vi "Test My JKI State Machine API.vi"() -> ()   [LabVIEW 2014, in "JKISM Example echo DQMH.lvlib"]
uses:
  JKISM Example echo DQMH.lvlib
  user.lib/_NEVSTOP/JKI State Machine ++/_Support/JKISMQ/_JKISMQFGV.vi
  user.lib/_NEVSTOP/JKI State Machine ++/JKI-State-Machine-Plus.lvlib
panel:
  out "Active Module":string[](array[string])
  in  "Select  Module":string(combo)
  out "Reply":string
  in  "X":dbl=1.0
  in  "wait for reply":bool=TRUE
  out "Reply Payload":dbl
  in  "Stop Module":bool
  in  "Start Module":bool
  in  "Test Do Something Else and Wait for Reply":bool
  in  "Hide Module Panel":bool
  in  "Show Module Panel":bool
  in  "Test Do Something Else":bool
  in  "Test Do Something":bool
  # "1. Support both Singleton and Cloneable , compare with DQMH Template\n2. Use the reply method -> as the replacement of status report in DQMH Template"
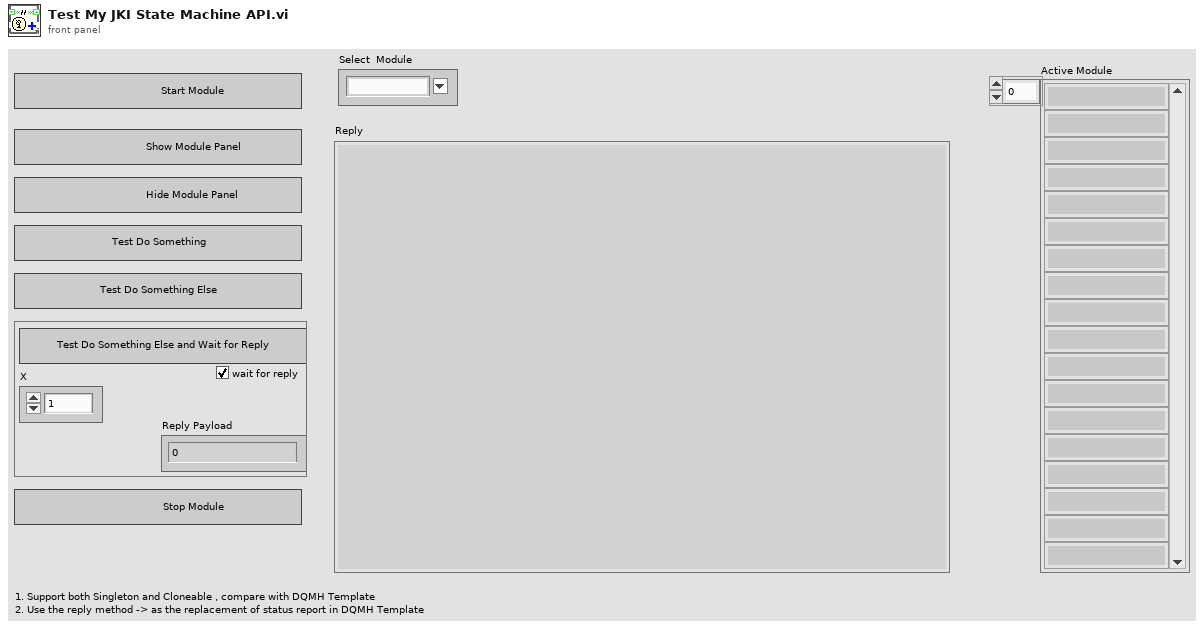
[diagram p1: front panel]
types:
  T1 = enum32{"Invalid", "Standard", "Closed", "Hidden", "Minimized", "Maximized"}
  T2 = enum32{"invalid app kind", "Development System", "Run Time System", "Student Edition", "Embedded LabVIEW", "Evaluation", "Custom"}
  T3 = cluster{"Core":cluster{"Current VI Reference":refnum<vi>, "Close Panel on Exit?":bool}, "Your Boolean data":bool, "Your string data":string, "Select  Module":refnum<vi>}
  T4 = cluster{"Current VI Reference":refnum<vi>, "Close Panel on Exit?":bool}
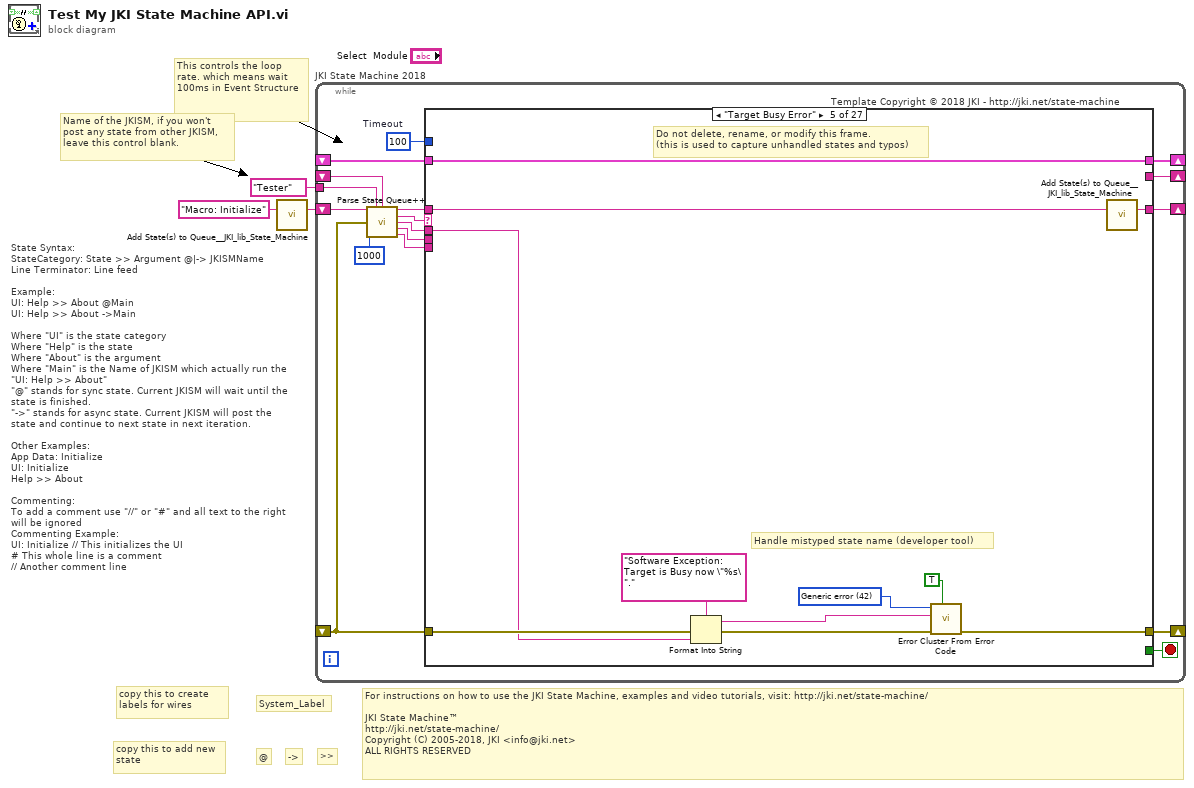
[diagram p0: block diagram]
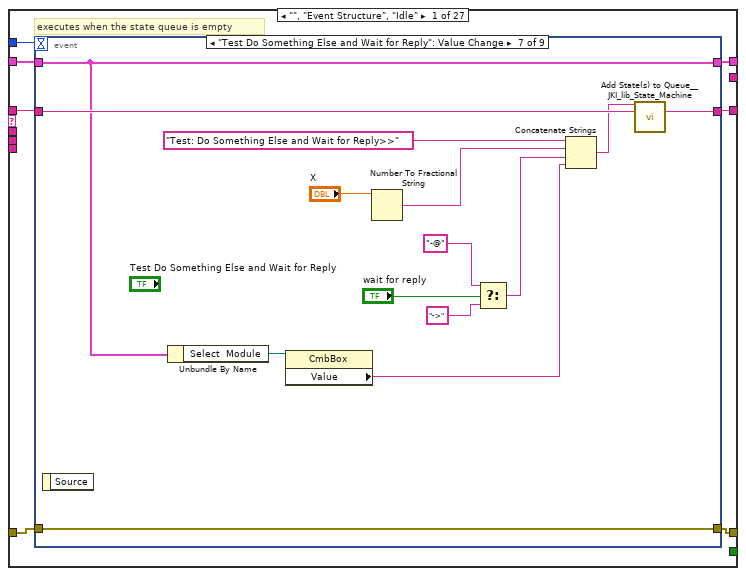
[diagram p2: hidden frame]
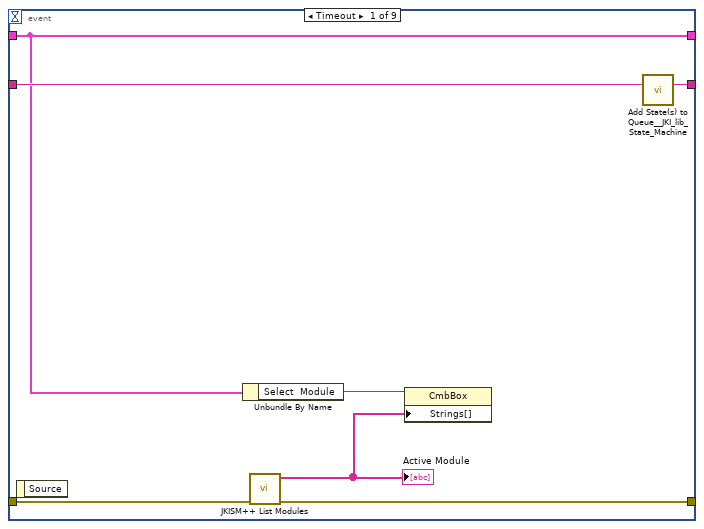
[diagram p3: hidden frame]
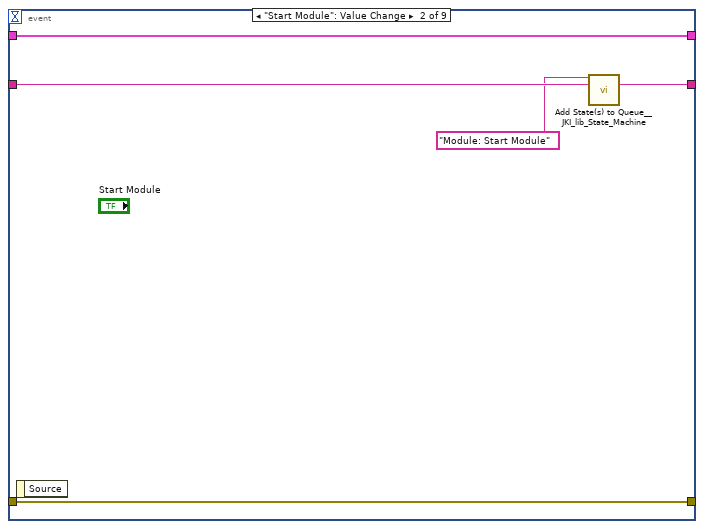
[diagram p4: hidden frame]
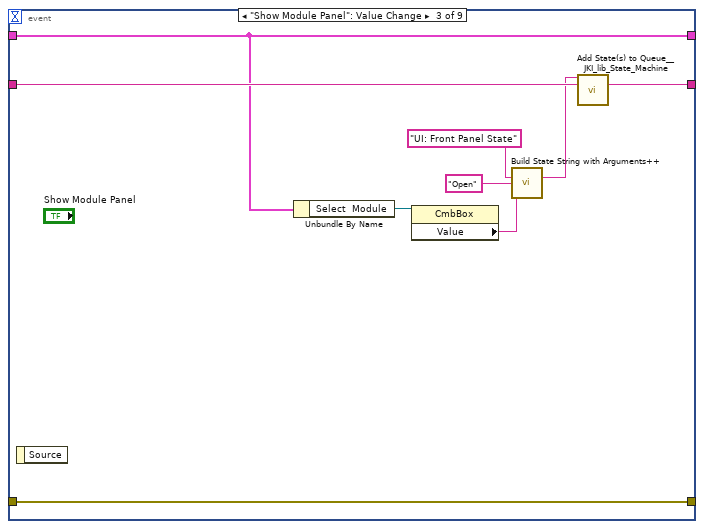
[diagram p5: hidden frame]
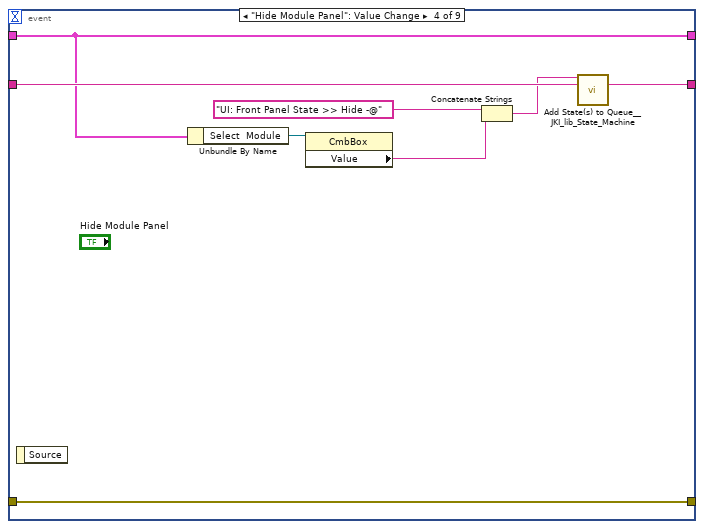
[diagram p6: hidden frame]
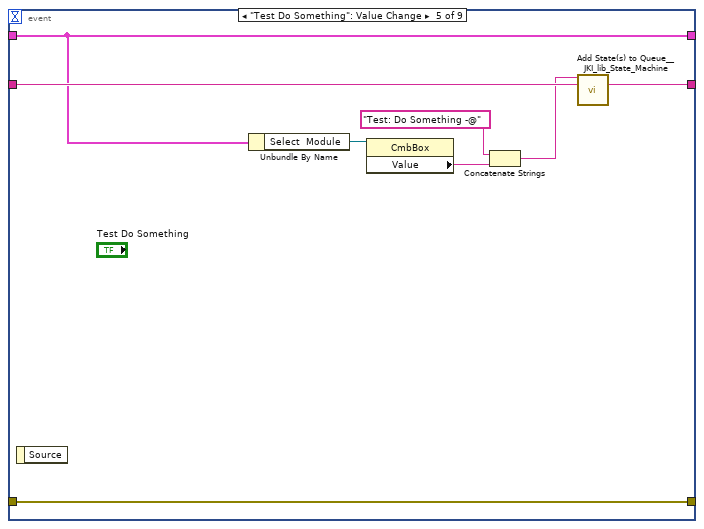
[diagram p7: hidden frame]
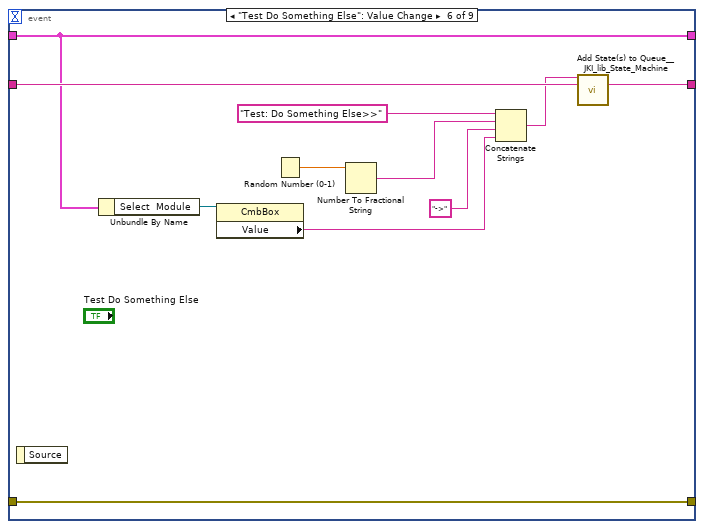
[diagram p8: hidden frame]
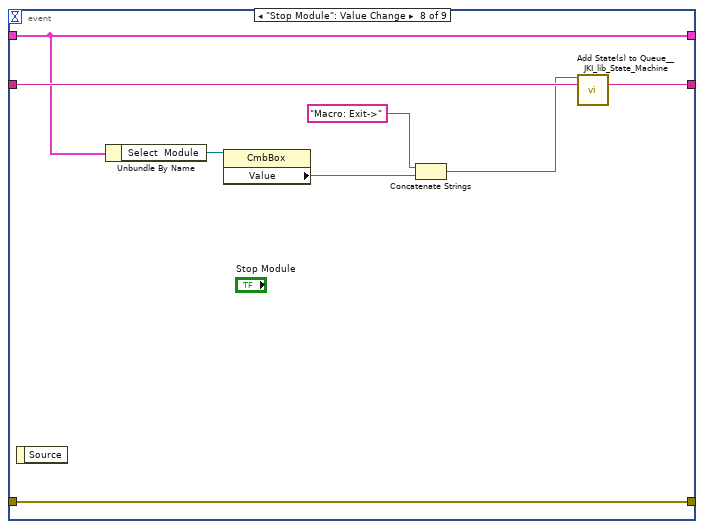
[diagram p9: hidden frame]
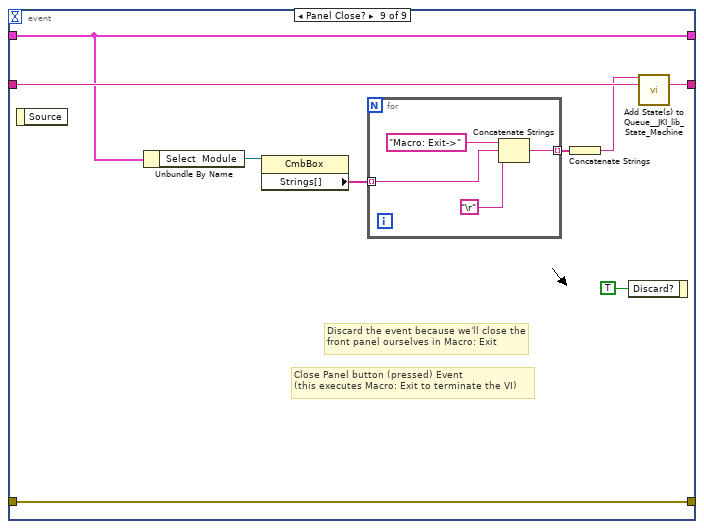
[diagram p10: hidden frame]
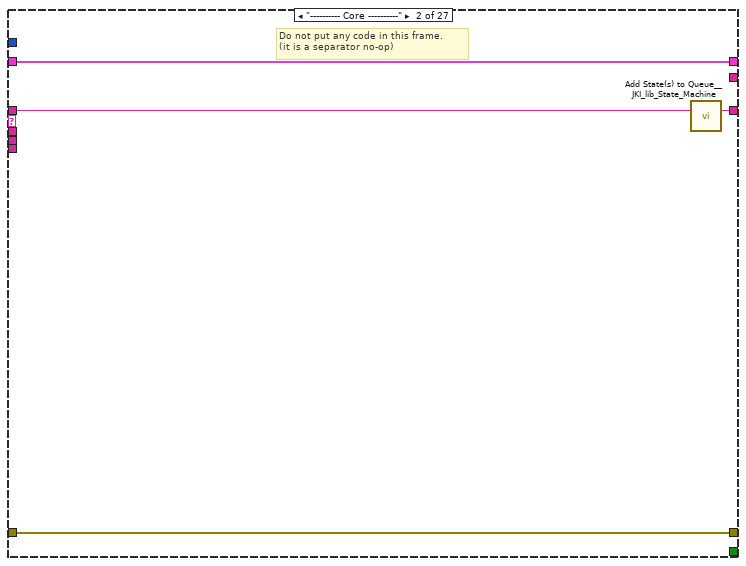
[diagram p11: hidden frame]
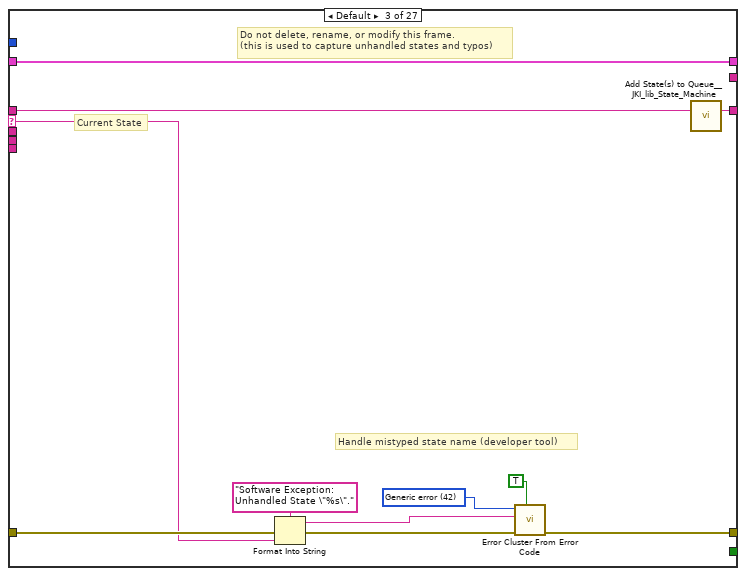
[diagram p12: hidden frame]
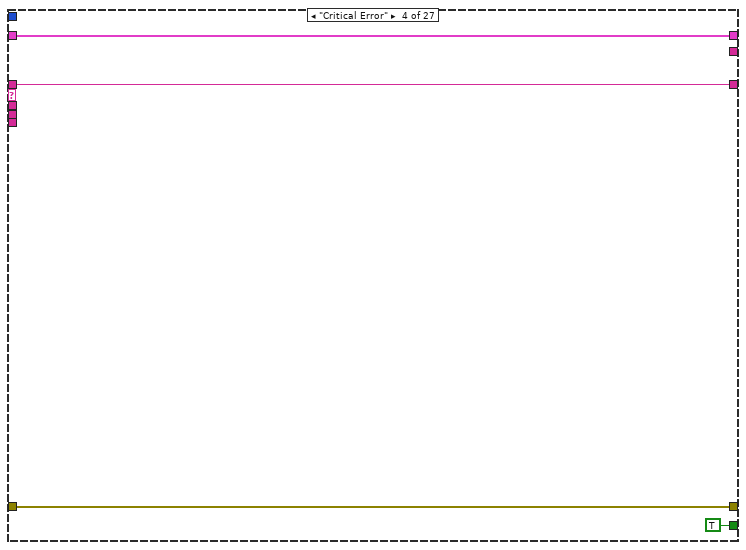
[diagram p13: hidden frame]
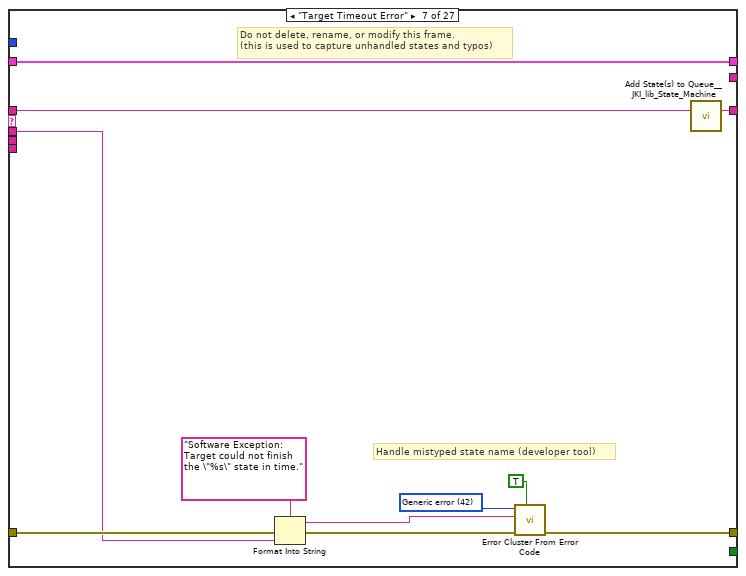
[diagram p15: hidden frame]
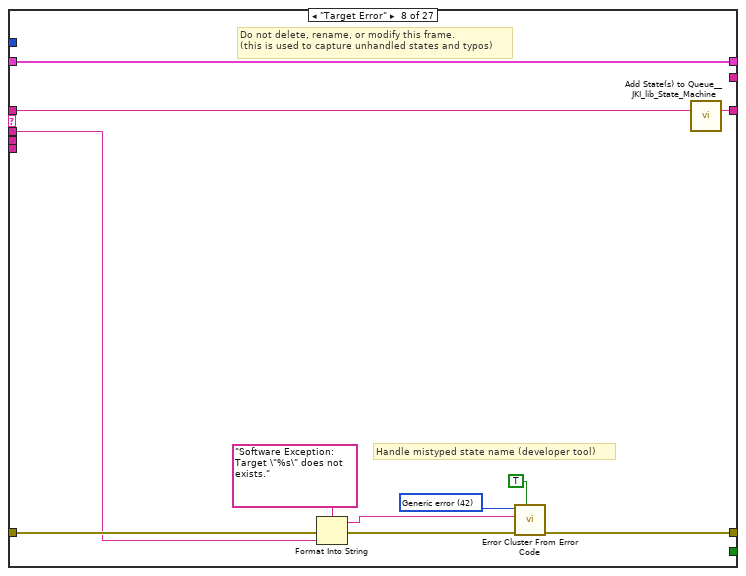
[diagram p16: hidden frame]
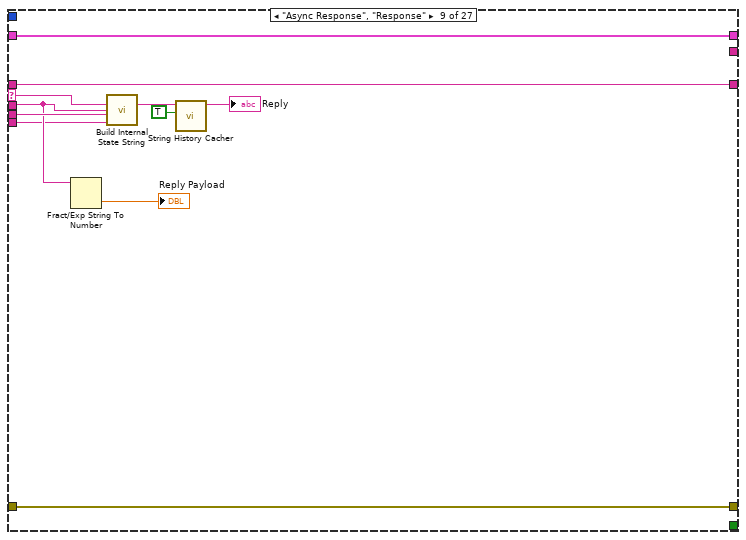
[diagram p17: hidden frame]
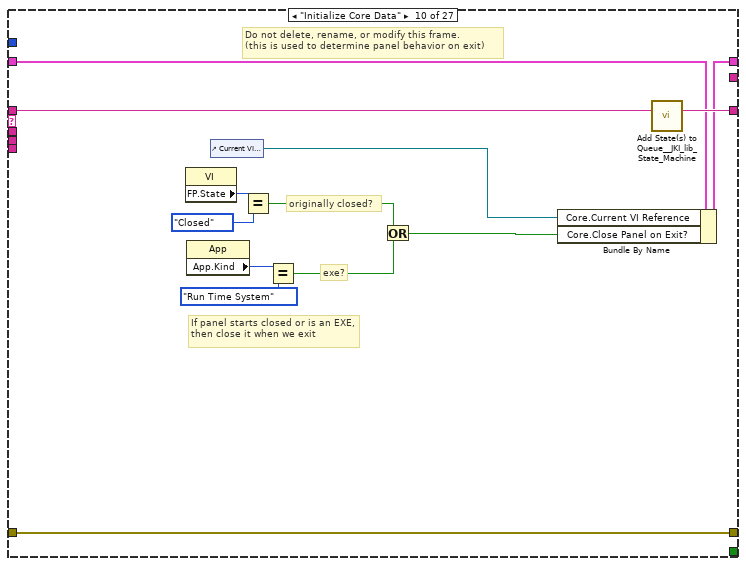
[diagram p18: hidden frame]
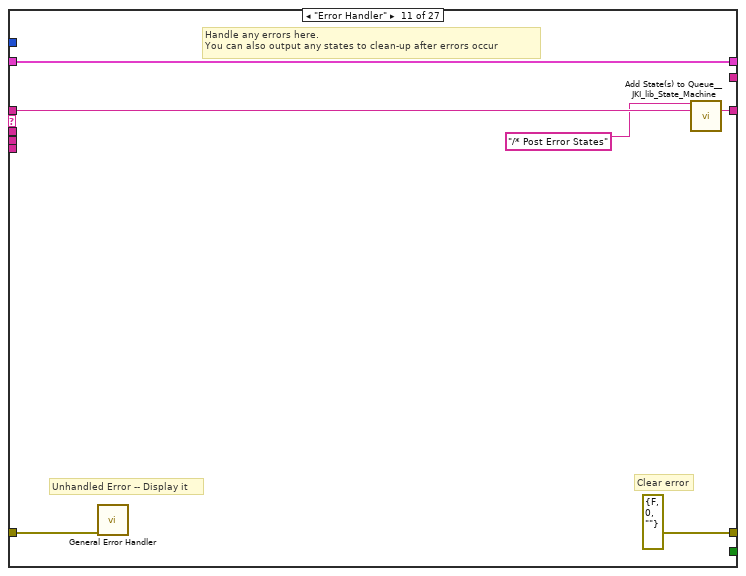
[diagram p19: hidden frame]
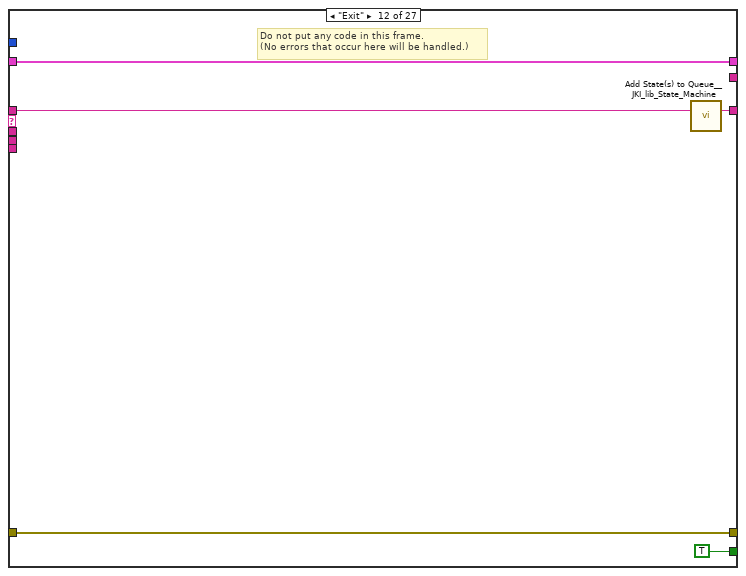
[diagram p20: hidden frame]
diagram:
  # "copy this to add new state"
  # ">>"
  # "->"
  # "@"
  # "Name of the JKISM, if you won't post any state from other JKISM,  leave this control blank."
  # "For instructions on how to use the JKI State Machine, examples and video tutorials, visit: http://jki.net/state-machine/\n\nJKI State Machine™\nhttp://jki.net/state-machine/\nCopyright (C) 2005-2018, JKI <info@jki.net>\nALL RIGHTS RESERVED"
  # "State Syntax:\nStateCategory: State >> Argument @|-> JKISMName\nLine Terminator: Line feed\n\nExample:\nUI: Help >> About @Main\nUI: Help >> About ->Main\n\nWhere \"UI\" is the state category\nWhere \"Help\" is the state\nWhere \"About\" is the argument\nWhere \"Main\" is the Name of JKISM which actually run the \"UI: Help >> About\"\n\"@\" stands for sync state. Current JKISM will wait until the state is finished.\n\"->\" stands for async state. Current JKISM will post the state and continue to next state in next iteration.\n\nOther Examples:\nApp Data: Initialize\nUI: Initialize\nHelp >> About\n\nCommenting:\nTo add a comment use \"//\" or \"#\" and all text to the right will be ignored\nCommenting Example:\nUI: Initialize // This initializes the UI\n# This whole line is a comment\n// Another comment line"
  # "copy this to create labels for wires"
  # "This controls the loop rate. which means wait 100ms in Event Structure"
  # "System_Label"
  n1 = call <vilib>:"Add State(s) to Queue__JKI_lib_State_Machine.vi"("State(s) in (\"\")"="Macro: Initialize") -> ("States Out"=w3:string)  [unwired: 14 in]
  n2 = while "JKI State Machine 2018" {
    shift-right: [w15] -> _
    shift-left: _ -> [w14]
    shift-right: [w18] -> _
    shift-left: _ -> [w12]
    shift-right: [w17] -> _
    shift-left: w3 -> [w19]
    tunnel: "Tester" ("Name(\"\" to use uuid)") -> [w8]
    shift-right: [w4] -> _
    shift-left: _ -> [w5]
    stop <- w16 stop-if-true
    w13 = 100  # Timeout
    # "Template Copyright © 2018 JKI - http://jki.net/state-machine"
    n3 = call "Parse State Queue++.vi"("State Queue"=w19, "Name(\"\" to use uuid)"=w8, "Response Arguments"=w5, "Error In (no error)"=w12, "Response Timeout(5000ms)"=1000 ("Response Timeout(1000ms)")) -> ("Remaining States"=w20:string, "Current State"=w11:string, "Arguments"=w10:string, "Argument - State"=w6:string, "From Who"=w9:string)  [unwired: 5 in, 1 out]
    n4 = case shown="\"Target Busy Error\"" w11 {
      selector: w11 -> [_ _ w115 _ _ _ _ _ w173 _ _ _ _ _ _ _ _ _ _ _ _ _ _ _ _ _ _]
      tunnel: w20 -> [w27 w114 w119 w128 w134 w142 w148 w159 w175 w189 w195 w200 w204 w212 w218 w222 w226 w232 w243 w312 w317 w327 w331 w335 w339 w341 w350]
      tunnel: w10 -> [_ _ _ _ w130 _ w144 w155 w169 _ _ _ _ _ _ _ _ w227 w237 _ _ _ _ _ _ _ _]
      tunnel: w14 -> [w25 w111 w117 w127 w132 w141 w146 w157 w174 w182 w192 w198 w201 _ w213 w219 w224 w230 w239 w309 w314 w324 w328 w332 w336 w340 w361]
      tunnel: [w24 w112 w121 w129 w136 w143 w150 w161 w176 w186 errorcluster {"status"=FALSE, "code"=0, "source"=""} ("error out") w197 w202 w209 w214 w220 w223 w228 w240 w310 w315 w325 w329 w333 w337 w342 w349] -> w18
      tunnel: w12 -> [w23 w112 w120 w129 w135 w143 w149 w160 w176 w186 w191 w197 w202 w209 w215 w220 w223 w229 w241 w310 w315 w325 w329 w333 w337 w342 w359]
      tunnel: [w26 w113 w118 w128 w133 w142 w147 w158 w175 w188 w194 w199 w203 w211 w217 w221 w225 w231 w242 w311 w316 w326 w330 w334 w338 w341 w350] -> w17
      tunnel: [_ _ _ TRUE _ _ _ _ _ _ _ TRUE _ _ _ _ _ _ _ _ _ _ _ _ _ _ _] -> w16
      tunnel: [w22 w111 w117 w127 w132 w141 w146 w157 w174 w187 w192 w198 w201 w210 w213 w219 w224 w230 w239 w309 w314 w324 w328 w332 w336 w340 w361] -> w15
      tunnel: w13 -> [w21 _ _ _ _ _ _ _ _ _ _ _ _ _ _ _ _ _ _ _ _ _ _ _ _ _ _]
      tunnel: w9 -> [_ _ _ _ _ _ _ _ w167 _ _ _ _ _ _ _ _ _ _ _ _ _ _ _ _ _ _]
      tunnel: w6 -> [_ _ _ _ _ _ _ _ w172 _ _ _ _ _ _ _ _ _ _ _ _ _ _ _ _ _ _]
      tunnel: [_ _ _ _ _ _ _ _ _ _ _ _ _ _ _ _ _ _ _ _ _ _ _ _ _ _ w343] -> w4
      frame "", "Event Structure", "Idle" {
        # "executes when the state queue is empty"
        n5 = event shown="[6] \"Test Do Something Else and Wait for Reply\": Value Change" {
          selector: _ -> [_ _ _ _ _ _ _ _ _]
          dyn-events: _ -> [_ _ _ _ _ _ _ _ _]
          timeout: w21 -> [_ _ _ _ _ _ _ _ _]
          tunnel: w27 -> [w34 w38 w48 w56 w64 w75 w89 w97 w106]
          tunnel: [w33 w37 w47 w55 w63 w74 w88 w96 w105] -> w26
          tunnel: w25 -> [w29 w39 w45 w52 w60 w66 w77 w93 w101]
          tunnel: [w31 w36 w46 w54 w62 w73 w87 w95 w104] -> w24
          tunnel: w23 -> [w32 w36 w46 w54 w62 w73 w87 w95 w104]
          tunnel: [w29 w39 w45 w52 w60 w66 w77 w93 w101] -> w22
          event Timeout {
            n6 = event-data() -> ()  [unwired: 1 in, 1 out]
            n7 = Unbundle By Name(w29) -> ("Select  Module"=w28:refnum<vi>)
            n8 = call "JKISM++ List Modules.vi"("Error in"=w32) -> ("Error out"=w31:errorcluster, "Name"=w30:string[])  [unwired: 9 in]
            "Active Module" <- w30
            n9 = property class="CmbBox"(reference=w28, "Strings[]"=w30) -> ()  [unwired: 1 in, 2 out]
            n10 = call <vilib>:"Add State(s) to Queue__JKI_lib_State_Machine.vi"("State(s) in (\"\")"=w34) -> ("States Out"=w33:string)  [unwired: 14 in]
          }
          event "Start Module": Value Change {
            n11 = event-data() -> ()  [unwired: 1 in, 1 out]
            n12 = call <vilib>:"Add State(s) to Queue__JKI_lib_State_Machine.vi"("State(s) in Front (\"\")"="Module: Start Module" ("State(s) in Front (\"\")"), "State(s) in (\"\")"=w38) -> ("States Out"=w37:string)  [unwired: 13 in]
          }
          event "Show Module Panel": Value Change {
            n13 = event-data() -> ()  [unwired: 1 in, 1 out]
            n14 = Unbundle By Name(w45) -> ("Select  Module"=w44:refnum<vi>)
            n15 = property class="CmbBox"(reference=w44) -> ("Value"=w43:string)  [unwired: 1 in, 2 out]
            n16 = call "Build State String with Arguments++.vi"("State"="UI: Front Panel State" ("State(s) in Front (\"\")"), "Arguments (\"\")"="Open" ("Arguments (\"\")"), "Dest Module (\"\")"=w43) -> ("State with Arguments"=w40:string)  [unwired: 12 in]
            n17 = call <vilib>:"Add State(s) to Queue__JKI_lib_State_Machine.vi"("State(s) in Front (\"\")"=w40, "State(s) in (\"\")"=w48) -> ("States Out"=w47:string)  [unwired: 13 in]
          }
          event "Hide Module Panel": Value Change {
            n18 = event-data() -> ()  [unwired: 1 in, 1 out]
            n19 = Unbundle By Name(w52) -> ("Select  Module"=w53:refnum<vi>)
            n20 = property class="CmbBox"(reference=w53) -> ("Value"=w50:string)  [unwired: 1 in, 2 out]
            n21 = Concatenate Strings("UI: Front Panel State >> Hide -@" ("State(s) in Front (\"\")"), w50) -> (w49:string)
            n22 = call <vilib>:"Add State(s) to Queue__JKI_lib_State_Machine.vi"("State(s) in Front (\"\")"=w49, "State(s) in (\"\")"=w56) -> ("States Out"=w55:string)  [unwired: 13 in]
          }
          event "Test Do Something": Value Change {
            n23 = event-data() -> ()  [unwired: 1 in, 1 out]
            n24 = Unbundle By Name(w60) -> ("Select  Module"=w61:refnum<vi>)
            n25 = property class="CmbBox"(reference=w61) -> ("Value"=w59:string)  [unwired: 1 in, 2 out]
            n26 = Concatenate Strings("Test: Do Something -@" ("State(s) in Front (\"\")"), w59) -> (w57:string)
            n27 = call <vilib>:"Add State(s) to Queue__JKI_lib_State_Machine.vi"("State(s) in Front (\"\")"=w57, "State(s) in (\"\")"=w64) -> ("States Out"=w63:string)  [unwired: 13 in]
          }
          event "Test Do Something Else": Value Change {
            n28 = event-data() -> ()  [unwired: 1 in, 1 out]
            n29 = Unbundle By Name(w66) -> ("Select  Module"=w67:refnum<vi>)
            n30 = property class="CmbBox"(reference=w67) -> ("Value"=w65:string)  [unwired: 1 in, 2 out]
            n31 = Random Number (0-1)() -> (number: 0 to 1=w72:dbl)
            n32 = Number To Fractional String(number=w72) -> (F-format string=w70:string)  [unwired: 3 in]
            n33 = Concatenate Strings("Test: Do Something Else>>" ("State(s) in Front (\"\")"), w70, "->" ("string"), w65) -> (w68:string)
            n34 = call <vilib>:"Add State(s) to Queue__JKI_lib_State_Machine.vi"("State(s) in Front (\"\")"=w68, "State(s) in (\"\")"=w75) -> ("States Out"=w74:string)  [unwired: 13 in]
          }
          event "Test Do Something Else and Wait for Reply": Value Change {
            n35 = event-data() -> ()  [unwired: 1 in, 1 out]
            n36 = Unbundle By Name(w77) -> ("Select  Module"=w78:refnum<vi>)
            n37 = property class="CmbBox"(reference=w78) -> ("Value"=w76:string)  [unwired: 1 in, 2 out]
            n38 = Number To Fractional String(number="X") -> (F-format string=w85:string)  [unwired: 3 in]
            n39 = Select(t="-@" ("string"), s="wait for reply", f="->" ("string")) -> (s? t:f=w80:string)
            n40 = Concatenate Strings("Test: Do Something Else and Wait for Reply>>" ("State(s) in Front (\"\")"), w85, w80, w76) -> (w84:string)
            n41 = call <vilib>:"Add State(s) to Queue__JKI_lib_State_Machine.vi"("State(s) in Front (\"\")"=w84, "State(s) in (\"\")"=w89) -> ("States Out"=w88:string)  [unwired: 13 in]
          }
          event "Stop Module": Value Change {
            n42 = event-data() -> ()  [unwired: 1 in, 1 out]
            n43 = Unbundle By Name(w93) -> ("Select  Module"=w94:refnum<vi>)
            n44 = property class="CmbBox"(reference=w94) -> ("Value"=w92:string)  [unwired: 1 in, 2 out]
            n45 = Concatenate Strings("Macro: Exit->" ("State(s) in Front (\"\")"), w92) -> (w90:string)
            n46 = call <vilib>:"Add State(s) to Queue__JKI_lib_State_Machine.vi"("State(s) in Front (\"\")"=w90, "State(s) in (\"\")"=w97) -> ("States Out"=w96:string)  [unwired: 13 in]
          }
          event Panel Close? {
            # "Discard the event because we'll close the front panel ourselves in Macro: Exit"
            # "Close Panel button (pressed) Event\n(this executes Macro: Exit to terminate the VI)"
            n47 = event-data() -> ()  [unwired: 1 in, 1 out]
            n48 = Unbundle By Name(w101) -> ("Select  Module"=w102:refnum<vi>)
            n49 = property class="CmbBox"(reference=w102) -> ("Strings[]"=w100:string[])  [unwired: 1 in, 2 out]
            n50 = for {
              tunnel: w100 -> [w109] mode=indexing
              tunnel: [w108] -> w99 mode=indexing
              n51 = Concatenate Strings("Macro: Exit->", w109, "\r") -> (w108:string)
            }
            n52 = Concatenate Strings(w99) -> (w98:string)
            n53 = event-data("Discard?"=TRUE) -> ()  [unwired: 1 in, 1 out]
            n54 = call <vilib>:"Add State(s) to Queue__JKI_lib_State_Machine.vi"("State(s) in Front (\"\")"=w98, "State(s) in (\"\")"=w106) -> ("States Out"=w105:string)  [unwired: 13 in]
          }
        }
      }
      frame "---------- Core ----------" {
        # "Do not put any code in this frame.\n(it is a separator no-op)"
        n55 = call <vilib>:"Add State(s) to Queue__JKI_lib_State_Machine.vi"("State(s) in (\"\")"=w114) -> ("States Out"=w113:string)  [unwired: 14 in]
      }
      frame Default {
        w124 = 42 items=["No error", "Argument error", "Memory is full", "Out of zone", "End of file", "File already open", "Generic file I/O error", "File not found", "File permission error", "Disk is full", "Duplicate path", "Too many files open", "System feature not enabled", "Resource file not found", "Cannot add resource", "Resource not found", "Image not found", "Image memory error", "Pen does not exist", "Config type invalid", "Config token not found", "Config parse error", "Config memory error", "Bad external code format", "Bad external code offset", "External code not present", "Null window", "Destroy window error", "Null menu", "Print aborted", "Bad print record", "Print driver error", "Windows error during printing", "Memory error during printing", "Print dialog error", "Generic print error", "Invalid device refnum", "Device not found", "Device parameter error", "Device unit error", "Cannot open device", "Device call aborted", "Generic error", "Cancelled by user", "Object ID too low", "Object ID too high", "Object not in heap", "Unknown heap", "Unknown object (invalid DefProc)", "Unknown object (DefProc not in table)", "Message out of range", "Invalid (null) method", "Unknown message", "Manager call not supported", "Bad address", "Network operation in progress", "Network operation timed out", "Connection is busy", "Network attribute not supported", "Network error", "Address in use", "System out of memory", "Connection aborted", "Connection refused", "Not connected", "Already connected", "Connection closed", "Initialization error (interapplication manager)", "Bad occurrence", "Wait on unbound occurrence handler", "Occurrence queue overflow", "Datalog type conflict", "Unused", "Unrecognized type (interapplication manager)", "Memory corrupt", "Failed to make temporary DLL", "Old CIN version", "Drag socket not found", "Failed to load drop-object", "Failed to register OLE object", "Failed to release OLE object", "Format specifier type mismatch", "Unknown format specifier", "Too few format specifiers", "Too many format specifiers", "Scan failed", "Newer CIN version", "Error converting to variant", "Runtime menu error", "Password tampered", "Variant attribute not found", "Incompatible variant data type", "Event data is not available", "Event Store is not present", "Occurrence is not found", "Event Queue is not created", "Event info is not available", "Refnum passed is NULL", "Error retrieving Class GUID", "Error retrieving CoClass GUID", "Error retrieving TypeLib GUID.", "Bad built application magic bytes.", "Specific driver is different from the specific driver associated with the Logical Name.", "There is no session opened to the class driver.", "Max Error", "MAX - Error with config objects", "MAX - Error loading configuration", "MAX - Group not supported"]
        # "Current State"
        # "Do not delete, rename, or modify this frame.\n(this is used to capture unhandled states and typos)"
        # "Handle mistyped state name (developer tool)"
        n56 = Format Into String(format string="Software Exception: Unhandled State \"%s\"." ("message"), error in=w120, w115) -> (resulting string=w123:string, error out=w122:errorcluster)  [unwired: 1 in]
        n57 = call <vilib>:"Error Cluster From Error Code.vi"("show call chain? (False)"=TRUE, "error in (no error)"=w122, "error message (\"\")"=w123, "error code (0)"=w124) -> ("error out"=w121:errorcluster)  [unwired: 5 in]
        n58 = call <vilib>:"Add State(s) to Queue__JKI_lib_State_Machine.vi"("State(s) in (\"\")"=w119) -> ("States Out"=w118:string)  [unwired: 14 in]
      }
      frame "Critical Error" {
      }
      frame "Target Busy Error" {
        w139 = 42 items=["No error", "Argument error", "Memory is full", "Out of zone", "End of file", "File already open", "Generic file I/O error", "File not found", "File permission error", "Disk is full", "Duplicate path", "Too many files open", "System feature not enabled", "Resource file not found", "Cannot add resource", "Resource not found", "Image not found", "Image memory error", "Pen does not exist", "Config type invalid", "Config token not found", "Config parse error", "Config memory error", "Bad external code format", "Bad external code offset", "External code not present", "Null window", "Destroy window error", "Null menu", "Print aborted", "Bad print record", "Print driver error", "Windows error during printing", "Memory error during printing", "Print dialog error", "Generic print error", "Invalid device refnum", "Device not found", "Device parameter error", "Device unit error", "Cannot open device", "Device call aborted", "Generic error", "Cancelled by user", "Object ID too low", "Object ID too high", "Object not in heap", "Unknown heap", "Unknown object (invalid DefProc)", "Unknown object (DefProc not in table)", "Message out of range", "Invalid (null) method", "Unknown message", "Manager call not supported", "Bad address", "Network operation in progress", "Network operation timed out", "Connection is busy", "Network attribute not supported", "Network error", "Address in use", "System out of memory", "Connection aborted", "Connection refused", "Not connected", "Already connected", "Connection closed", "Initialization error (interapplication manager)", "Bad occurrence", "Wait on unbound occurrence handler", "Occurrence queue overflow", "Datalog type conflict", "Unused", "Unrecognized type (interapplication manager)", "Memory corrupt", "Failed to make temporary DLL", "Old CIN version", "Drag socket not found", "Failed to load drop-object", "Failed to register OLE object", "Failed to release OLE object", "Format specifier type mismatch", "Unknown format specifier", "Too few format specifiers", "Too many format specifiers", "Scan failed", "Newer CIN version", "Error converting to variant", "Runtime menu error", "Password tampered", "Variant attribute not found", "Incompatible variant data type", "Event data is not available", "Event Store is not present", "Occurrence is not found", "Event Queue is not created", "Event info is not available", "Refnum passed is NULL", "Error retrieving Class GUID", "Error retrieving CoClass GUID", "Error retrieving TypeLib GUID.", "Bad built application magic bytes.", "Specific driver is different from the specific driver associated with the Logical Name.", "There is no session opened to the class driver.", "Max Error", "MAX - Error with config objects", "MAX - Error loading configuration", "MAX - Group not supported"]
        # "Do not delete, rename, or modify this frame.\n(this is used to capture unhandled states and typos)"
        # "Handle mistyped state name (developer tool)"
        n59 = Format Into String(format string="Software Exception: Target is Busy now \"%s\"." ("message"), error in=w135, w130) -> (resulting string=w138:string, error out=w137:errorcluster)  [unwired: 1 in]
        n60 = call <vilib>:"Error Cluster From Error Code.vi"("show call chain? (False)"=TRUE, "error in (no error)"=w137, "error message (\"\")"=w138, "error code (0)"=w139) -> ("error out"=w136:errorcluster)  [unwired: 5 in]
        n61 = call <vilib>:"Add State(s) to Queue__JKI_lib_State_Machine.vi"("State(s) in (\"\")"=w134) -> ("States Out"=w133:string)  [unwired: 14 in]
      }
      frame "Async Message Posted" {
      }
      frame "Target Timeout Error" {
        w153 = 42 items=["No error", "Argument error", "Memory is full", "Out of zone", "End of file", "File already open", "Generic file I/O error", "File not found", "File permission error", "Disk is full", "Duplicate path", "Too many files open", "System feature not enabled", "Resource file not found", "Cannot add resource", "Resource not found", "Image not found", "Image memory error", "Pen does not exist", "Config type invalid", "Config token not found", "Config parse error", "Config memory error", "Bad external code format", "Bad external code offset", "External code not present", "Null window", "Destroy window error", "Null menu", "Print aborted", "Bad print record", "Print driver error", "Windows error during printing", "Memory error during printing", "Print dialog error", "Generic print error", "Invalid device refnum", "Device not found", "Device parameter error", "Device unit error", "Cannot open device", "Device call aborted", "Generic error", "Cancelled by user", "Object ID too low", "Object ID too high", "Object not in heap", "Unknown heap", "Unknown object (invalid DefProc)", "Unknown object (DefProc not in table)", "Message out of range", "Invalid (null) method", "Unknown message", "Manager call not supported", "Bad address", "Network operation in progress", "Network operation timed out", "Connection is busy", "Network attribute not supported", "Network error", "Address in use", "System out of memory", "Connection aborted", "Connection refused", "Not connected", "Already connected", "Connection closed", "Initialization error (interapplication manager)", "Bad occurrence", "Wait on unbound occurrence handler", "Occurrence queue overflow", "Datalog type conflict", "Unused", "Unrecognized type (interapplication manager)", "Memory corrupt", "Failed to make temporary DLL", "Old CIN version", "Drag socket not found", "Failed to load drop-object", "Failed to register OLE object", "Failed to release OLE object", "Format specifier type mismatch", "Unknown format specifier", "Too few format specifiers", "Too many format specifiers", "Scan failed", "Newer CIN version", "Error converting to variant", "Runtime menu error", "Password tampered", "Variant attribute not found", "Incompatible variant data type", "Event data is not available", "Event Store is not present", "Occurrence is not found", "Event Queue is not created", "Event info is not available", "Refnum passed is NULL", "Error retrieving Class GUID", "Error retrieving CoClass GUID", "Error retrieving TypeLib GUID.", "Bad built application magic bytes.", "Specific driver is different from the specific driver associated with the Logical Name.", "There is no session opened to the class driver.", "Max Error", "MAX - Error with config objects", "MAX - Error loading configuration", "MAX - Group not supported"]
        # "Do not delete, rename, or modify this frame.\n(this is used to capture unhandled states and typos)"
        # "Handle mistyped state name (developer tool)"
        n62 = Format Into String(format string="Software Exception: Target could not finish the \"%s\" state in time." ("message"), error in=w149, w144) -> (resulting string=w152:string, error out=w151:errorcluster)  [unwired: 1 in]
        n63 = call <vilib>:"Error Cluster From Error Code.vi"("show call chain? (False)"=TRUE, "error in (no error)"=w151, "error message (\"\")"=w152, "error code (0)"=w153) -> ("error out"=w150:errorcluster)  [unwired: 5 in]
        n64 = call <vilib>:"Add State(s) to Queue__JKI_lib_State_Machine.vi"("State(s) in (\"\")"=w148) -> ("States Out"=w147:string)  [unwired: 14 in]
      }
      frame "Target Error" {
        w164 = 42 items=["No error", "Argument error", "Memory is full", "Out of zone", "End of file", "File already open", "Generic file I/O error", "File not found", "File permission error", "Disk is full", "Duplicate path", "Too many files open", "System feature not enabled", "Resource file not found", "Cannot add resource", "Resource not found", "Image not found", "Image memory error", "Pen does not exist", "Config type invalid", "Config token not found", "Config parse error", "Config memory error", "Bad external code format", "Bad external code offset", "External code not present", "Null window", "Destroy window error", "Null menu", "Print aborted", "Bad print record", "Print driver error", "Windows error during printing", "Memory error during printing", "Print dialog error", "Generic print error", "Invalid device refnum", "Device not found", "Device parameter error", "Device unit error", "Cannot open device", "Device call aborted", "Generic error", "Cancelled by user", "Object ID too low", "Object ID too high", "Object not in heap", "Unknown heap", "Unknown object (invalid DefProc)", "Unknown object (DefProc not in table)", "Message out of range", "Invalid (null) method", "Unknown message", "Manager call not supported", "Bad address", "Network operation in progress", "Network operation timed out", "Connection is busy", "Network attribute not supported", "Network error", "Address in use", "System out of memory", "Connection aborted", "Connection refused", "Not connected", "Already connected", "Connection closed", "Initialization error (interapplication manager)", "Bad occurrence", "Wait on unbound occurrence handler", "Occurrence queue overflow", "Datalog type conflict", "Unused", "Unrecognized type (interapplication manager)", "Memory corrupt", "Failed to make temporary DLL", "Old CIN version", "Drag socket not found", "Failed to load drop-object", "Failed to register OLE object", "Failed to release OLE object", "Format specifier type mismatch", "Unknown format specifier", "Too few format specifiers", "Too many format specifiers", "Scan failed", "Newer CIN version", "Error converting to variant", "Runtime menu error", "Password tampered", "Variant attribute not found", "Incompatible variant data type", "Event data is not available", "Event Store is not present", "Occurrence is not found", "Event Queue is not created", "Event info is not available", "Refnum passed is NULL", "Error retrieving Class GUID", "Error retrieving CoClass GUID", "Error retrieving TypeLib GUID.", "Bad built application magic bytes.", "Specific driver is different from the specific driver associated with the Logical Name.", "There is no session opened to the class driver.", "Max Error", "MAX - Error with config objects", "MAX - Error loading configuration", "MAX - Group not supported"]
        # "Do not delete, rename, or modify this frame.\n(this is used to capture unhandled states and typos)"
        # "Handle mistyped state name (developer tool)"
        n65 = Format Into String(format string="Software Exception: Target \"%s\" does not exists." ("message"), error in=w160, w155) -> (resulting string=w163:string, error out=w162:errorcluster)  [unwired: 1 in]
        n66 = call <vilib>:"Error Cluster From Error Code.vi"("show call chain? (False)"=TRUE, "error in (no error)"=w162, "error message (\"\")"=w163, "error code (0)"=w164) -> ("error out"=w161:errorcluster)  [unwired: 5 in]
        n67 = call <vilib>:"Add State(s) to Queue__JKI_lib_State_Machine.vi"("State(s) in (\"\")"=w159) -> ("States Out"=w158:string)  [unwired: 14 in]
      }
      frame "Async Response", "Response" {
        n68 = Fract/Exp String To Number(string=w169) -> (number=→"Reply Payload":dbl)  [unwired: 3 in, 1 out]
        n69 = call "Build Internal State String.vi"("State"=w173, "Arguments (\"\")"=w169, "Arg-State (\"\")"=w172, "Source (\"\")"=w167) -> ("State with Arguments"=w171:string)  [unwired: 11 in]
        n70 = call "String History Cacher.vi"("Include Timestamp(F)"=TRUE, "String"=w171) -> ("String Cache"=→"Reply":string)  [unwired: 9 in]
      }
      frame "Initialize Core Data" {
        # "Do not delete, rename, or modify this frame.\n(this is used to determine panel behavior on exit)"
        # "originally closed?"
        # "exe?"
        # "If panel starts closed or is an EXE, then close it when we exit"
        n71 = property class="VI"() -> ("FP.State"=w179:T1)  [unwired: 2 in, 2 out]
        n72 = property class="App"() -> ("App.Kind"=w185:T2)  [unwired: 2 in, 2 out]
        n73 = control-ref of="Current VI Reference"() -> (w180:refnum<vi>)
        n74 = Equal?(x=w179, y=T1."Closed" ("Front Panel Window:State")) -> (x = y?=w177:bool)
        n75 = Equal?(x=w185, y=T2."Run Time System" ("Application:Kind")) -> (x = y?=w183:bool)
        n76 = Or(x=w177, y=w183) -> (x .or. y?=w181:bool)
        n77 = Bundle By Name(cluster=w182, "Core.Current VI Reference"=w180, "Core.Close Panel on Exit?"=w181) -> (w187:T3)
        n78 = call <vilib>:"Add State(s) to Queue__JKI_lib_State_Machine.vi"("State(s) in (\"\")"=w189) -> ("States Out"=w188:string)  [unwired: 14 in]
      }
      frame "Error Handler" {
        # "Unhandled Error -- Display it"
        # "Handle any errors here.\nYou can also output any states to clean-up after errors occur"
        # "Clear error"
        n79 = call <vilib>:"General Error Handler.vi"("error in (no error)"=w191) -> ()  [unwired: 10 in, 5 out]
        n80 = call <vilib>:"Add State(s) to Queue__JKI_lib_State_Machine.vi"("State(s) in Front (\"\")"="/* Post Error States", "State(s) in (\"\")"=w195) -> ("States Out"=w194:string)  [unwired: 13 in]
      }
      frame "Exit" {
        # "Do not put any code in this frame.\n(No errors that occur here will be handled.)"
        n81 = call <vilib>:"Add State(s) to Queue__JKI_lib_State_Machine.vi"("State(s) in (\"\")"=w200) -> ("States Out"=w199:string)  [unwired: 14 in]
      }
      frame "---------- Data ----------" {
        # "Do not put any code in this frame.\n(It is a separator no-op. You can make a copy of this frame to create a new Data frame)"
        n82 = call <vilib>:"Add State(s) to Queue__JKI_lib_State_Machine.vi"("State(s) in (\"\")"=w204) -> ("States Out"=w203:string)  [unwired: 14 in]
      }
      frame "Data: Initialize" {
        w206 = T4 {"Current VI Reference"=refnum, "Close Panel on Exit?"=FALSE}  # Core
        w208 = TRUE  # Your Boolean data
        w207 = ""  # Your string data
        # "do not delete - used by framework"
        # "Expand Bundle to add new data elements to shift register data."
        # "Add new data here."
        # "Data names and types of shift register data are defined by this bundle."
        # "Initialize the shift-register data, here.\n(data names are defined by what you wire into the bundle function)"
        n83 = control-ref of="Select  Module"() -> (w205:refnum<vi>)
        n84 = Bundle("Core"=w206, "Your Boolean data"=w208, "Your string data"=w207, "Select  Module"=w205) -> (w210:T3)  [unwired: 1 in]
        n85 = call <vilib>:"Add State(s) to Queue__JKI_lib_State_Machine.vi"("State(s) in (\"\")"=w212) -> ("States Out"=w211:string)  [unwired: 14 in]
      }
      frame "Data: Cleanup" {
        # "Cleanup any data and references, here.\n(this is called automatically, by the Macro: Exit)"
        n86 = Unbundle By Name(w213) -> ("Core.Current VI Reference"=w216:refnum<vi>)
        n87 = Close Reference(reference=w216, error in (no error)=w215) -> (error out=w214:errorcluster)
        n88 = call <vilib>:"Add State(s) to Queue__JKI_lib_State_Machine.vi"("State(s) in (\"\")"=w218) -> ("States Out"=w217:string)  [unwired: 14 in]
      }
      frame "---------- UI ----------" {
        # "Do not put any code in this frame.\n(It is a separator no-op. You can make a copy of this frame to create a new UI frame)"
        n89 = call <vilib>:"Add State(s) to Queue__JKI_lib_State_Machine.vi"("State(s) in (\"\")"=w222) -> ("States Out"=w221:string)  [unwired: 14 in]
      }
      frame "UI: Initialize" {
        # "Initialize the User Interface, here.\n(this is called automatically, by the Macro: Init)"
        n90 = call <vilib>:"Add State(s) to Queue__JKI_lib_State_Machine.vi"("State(s) in (\"\")"=w226) -> ("States Out"=w225:string)  [unwired: 14 in]
      }
      frame "UI: Cursor Set" {
        # "Argument"
        # "Set and Unset Cursor Busy.\n(Usage: \"UI: Cursor Set >> Busy|Idle\")"
        n91 = case shown="\"Idle\", Default" w227 {
          tunnel: w229 -> [w234 w236]
          tunnel: [w233 w235] -> w228
          frame "Idle", Default {
            n92 = call <vilib>:"Unset Busy.vi"("error in (no error)"=w234) -> ("error out"=w233:errorcluster)  [unwired: 10 in]
          }
          frame "Busy" {
            n93 = call <vilib>:"Set Busy.vi"("error in (no error)"=w236) -> ("error out"=w235:errorcluster)  [unwired: 9 in, 1 out]
          }
        }
        n94 = call <vilib>:"Add State(s) to Queue__JKI_lib_State_Machine.vi"("State(s) in (\"\")"=w232) -> ("States Out"=w231:string)  [unwired: 14 in]
      }
      frame "UI: Front Panel State" {
        # "Argument"
        # "Set Front Panel Open or Closed\n(Usage: \"UI: Front Panel State >> Open|Close\")"
        n95 = Unbundle By Name(w239) -> ("Core.Current VI Reference"=w238:refnum<vi>)
        n96 = case shown="\"Hidden\", \"Hide\"" w237 {
          tunnel: w241 -> [w249 w264 w275 w288 w301]
          tunnel: [w251 w265 w277 w290 w303] -> w240
          tunnel: w238 -> [w250 w262 w276 w289 w302]
          frame "Open", "Standard", Default {
            w244 = T1."Standard" ("State")
            n97 = property class="VI"(reference=w250, error in=w249) -> (reference out=w247:refnum<vi>, error out=w248:errorcluster, "FP.State"=w246:T1)
            n98 = Not Equal?(x=w246, y=w244) -> (x != y?=w245:bool)
            n99 = case shown="True" w245 {
              tunnel: [w255 w257] -> w251
              tunnel: w248 -> [w254 w257]
              tunnel: w247 -> [w253 _]
              tunnel: w244 -> [w252 _]
              frame True {
                n100 = invoke class="VI" method="FP.Open"(reference=w253, error in=w254, "Activate"=TRUE, "State"=w252) -> (error out=w255:errorcluster)  [unwired: 1 in, 4 out]
              }
              frame False {
              }
            }
          }
          frame "Close", "Closed" {
            n101 = property class="VI"(reference=w262, error in=w264) -> (reference out=w261:refnum<vi>, error out=w263:errorcluster, "FP.State"=w259:T1)
            n102 = Not Equal?(x=w259, y=T1."Closed" ("Front Panel Window:State")) -> (x != y?=w258:bool)
            n103 = case shown="True" w258 {
              tunnel: [w266 w269] -> w265
              tunnel: w263 -> [w266 w268]
              tunnel: w261 -> [_ w267]
              frame False {
              }
              frame True {
                n104 = invoke class="VI" method="FP.Close"(reference=w267, error in=w268) -> (error out=w269:errorcluster)  [unwired: 1 in, 2 out]
              }
            }
          }
          frame "Hidden", "Hide" {
            w270 = T1."Hidden" ("State")
            n105 = property class="VI"(reference=w276, error in=w275) -> (reference out=w273:refnum<vi>, error out=w274:errorcluster, "FP.State"=w272:T1)
            n106 = Not Equal?(x=w272, y=w270) -> (x != y?=w271:bool)
            n107 = case shown="True" w271 {
              tunnel: [w281 w282] -> w277
              tunnel: w274 -> [w280 w282]
              tunnel: w273 -> [w279 _]
              tunnel: w270 -> [w278 _]
              frame True {
                n108 = invoke class="VI" method="FP.Open"(reference=w279, error in=w280, "State"=w278) -> (error out=w281:errorcluster)  [unwired: 2 in, 4 out]
              }
              frame False {
              }
            }
          }
          frame "Minimize", "Minimized" {
            w283 = T1."Minimized" ("State")
            n109 = property class="VI"(reference=w289, error in=w288) -> (reference out=w286:refnum<vi>, error out=w287:errorcluster, "FP.State"=w285:T1)
            n110 = Not Equal?(x=w285, y=w283) -> (x != y?=w284:bool)
            n111 = case shown="True" w284 {
              tunnel: [w294 w295] -> w290
              tunnel: w287 -> [w293 w295]
              tunnel: w286 -> [w292 _]
              tunnel: w283 -> [w291 _]
              frame True {
                n112 = invoke class="VI" method="FP.Open"(reference=w292, error in=w293, "State"=w291) -> (error out=w294:errorcluster)  [unwired: 2 in, 4 out]
              }
              frame False {
              }
            }
          }
          frame "Maximize", "Maximized" {
            w296 = T1."Maximized" ("State")
            n113 = property class="VI"(reference=w302, error in=w301) -> (reference out=w299:refnum<vi>, error out=w300:errorcluster, "FP.State"=w298:T1)
            n114 = Not Equal?(x=w298, y=w296) -> (x != y?=w297:bool)
            n115 = case shown="True" w297 {
              tunnel: [w307 w308] -> w303
              tunnel: w300 -> [w306 w308]
              tunnel: w299 -> [w305 _]
              tunnel: w296 -> [w304 _]
              frame True {
                n116 = invoke class="VI" method="FP.Open"(reference=w305, error in=w306, "State"=w304) -> (error out=w307:errorcluster)  [unwired: 2 in, 4 out]
              }
              frame False {
              }
            }
          }
        }
        n117 = call <vilib>:"Add State(s) to Queue__JKI_lib_State_Machine.vi"("State(s) in (\"\")"=w243) -> ("States Out"=w242:string)  [unwired: 14 in]
      }
      frame "---------- Macro ----------" {
        # "Do not put any code in this frame.\n(It is a separator no-op. You can make a copy of this frame to create a new Macro frame)"
        n118 = call <vilib>:"Add State(s) to Queue__JKI_lib_State_Machine.vi"("State(s) in (\"\")"=w312) -> ("States Out"=w311:string)  [unwired: 14 in]
      }
      frame "Macro: Initialize" {
        w313 = "Data: Initialize\nInitialize Core Data\nUI: Initialize\nUI: Front Panel State >> Open"  # Data: Initialize Initialize Core Data UI: Initialize UI: Front Panel State >> Open
        # "Initialization Macro\n(This is called once, when the VI starts)"
        n119 = call <vilib>:"Add State(s) to Queue__JKI_lib_State_Machine.vi"("State(s) in Front (\"\")"=w313, "State(s) in (\"\")"=w317) -> ("States Out"=w316:string)  [unwired: 13 in]
      }
      frame "Macro: Exit" {
        # "Exit Macro\n(This is called once, when the VI exits)"
        n120 = Unbundle By Name(w324) -> ("Core.Close Panel on Exit?"=w323:bool)
        n121 = Select(t="UI: Front Panel State >> Close", s=w323, f="") -> (s? t:f=w320:string)
        n122 = call <vilib>:"Add State(s) to Queue__JKI_lib_State_Machine.vi"("State(s) in (\"\")"=w320, "State(s) at Back (\"\")"="Data: Cleanup\nExit") -> ("States Out"=w318:string)  [unwired: 13 in]
        n123 = call <vilib>:"Add State(s) to Queue__JKI_lib_State_Machine.vi"("State(s) in Front (\"\")"=w318, "State(s) in (\"\")"=w327) -> ("States Out"=w326:string)  [unwired: 13 in]
      }
      frame "---------- New Category ----------" {
        # "Template Separator\n(You can make a copy of, or modify, this frame)"
        n124 = call <vilib>:"Add State(s) to Queue__JKI_lib_State_Machine.vi"("State(s) in (\"\")"=w331) -> ("States Out"=w330:string)  [unwired: 14 in]
      }
      frame "New Category: 1" {
        # "Your code here.\n(You can make a copy of, or modify, this frame)"
        n125 = call <vilib>:"Add State(s) to Queue__JKI_lib_State_Machine.vi"("State(s) in (\"\")"=w335) -> ("States Out"=w334:string)  [unwired: 14 in]
      }
      frame "New Category: 2" {
        # "Your code here.\n(You can make a copy of, or modify, this frame)"
        n126 = call <vilib>:"Add State(s) to Queue__JKI_lib_State_Machine.vi"("State(s) in (\"\")"=w339) -> ("States Out"=w338:string)  [unwired: 14 in]
      }
      frame "---------- Module ----------" {
      }
      frame "Module: Start Module" {
        n127 = vi-ref "My JKI State Machine Module.vi"() -> (w360:refnum<vi>)
        n128 = property class="VI"(reference=w360, error in=w359) -> (error out=w358:errorcluster, "Path"=w357:path)  [unwired: 1 out]
        n129 = feedback #1(0) -> (w347:i32)
        n130 = Increment(x=w347) -> (x+1=w346:i32)
        n131 = feedback-in #1(w346) -> ()
        n132 = Open VI Reference(type specifier VI Refnum (for type only)=refnum<vi> refnum, vi path=w357, options=128, error in (no error)=w358) -> (vi reference=w354:refnum<vi>, error out=w353:errorcluster)  [unwired: 2 in]
        n133 = Number To Decimal String(number=w346) -> (decimal integer string=w345:string)  [unwired: 1 in]
        n134 = Concatenate Strings("M" ("Module Name"), w345) -> (w343:string)
        n135 = call-by-ref "Start Asynchronous Call"(reference=w354, error in=w353, "Module Name"=w343) -> (reference out=w351:refnum<vi>, error out=w352:errorcluster)  [unwired: 11 in]
        n136 = Close Reference(reference=w351, error in (no error)=w352) -> (error out=w349:errorcluster)
      }
    }
  }
